vi "Get_All_Remote_SV_by_IP.vi"(8 "error in (no error)":errorcluster, 9 "timeout (30 s)":i32=30, 11 "IP Address":string="127.0.0.1") -> (0 "error out":errorcluster, 3 "Processes":T1(array[cluster]))   [LabVIEW 2016, in "DSC Remote SV Access.lvlib"]
doc: "This VI gets all the shared variables from a remote target.\n\nCreated By:\nRyan Pacini\n11/31/11"
uses:
  DSC Remote SV Access.lvlib
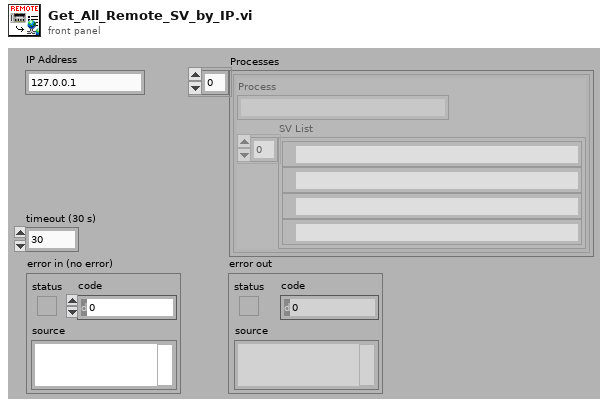
[diagram p1: front panel]
types:
  T1 = cluster{"Process":string, "SV List":refnum<k21>[]}[]
  T2 = cluster{string, "Shared Variable List":refnum<k21>[]}
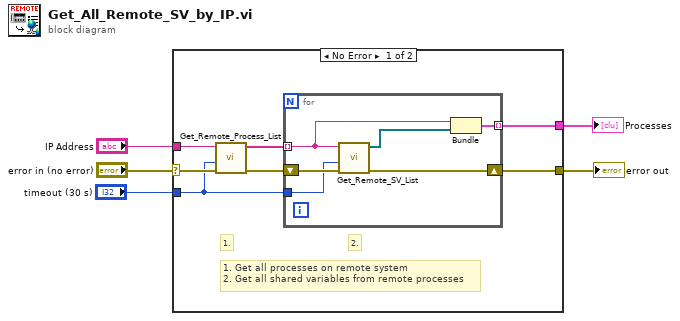
[diagram p0: block diagram]
diagram:
  n1 = case shown="No Error" "error in (no error)" {
    selector: "error in (no error)" -> [w7 w19]
    tunnel: [w10 _] -> w5
    tunnel: "IP Address" -> [w9 _]
    tunnel: [w8 w19] -> w3
    tunnel: "timeout (30 s)" -> [w6 _]
    frame No Error {
      # "1. Get all processes on remote system\n2. Get all shared variables from remote processes"
      # "2."
      # "1."
      n2 = call "Get_Remote_Process_List.vi"("error in (no error)"=w7, "timeout (30 s)"=w6, "IP Address"=w9) -> ("error out"=w12:errorcluster, "Process List (\\\\[IPAddress]\\[Process])"=w11:string[])  [unwired: 7 in]
      n3 = for {
        tunnel: w11 -> [w16] mode=indexing
        shift-right: [w17] -> w8
        shift-left: w12 -> [w18]
        tunnel: [w15] -> w10 mode=indexing
        tunnel: w6 -> [w14]
        n4 = call "Get_Remote_SV_List.vi"("error in (no error)"=w18, "timeout (30 s)"=w14, "Process (\\\\[IPAddress]\\[Process])"=w16) -> ("error out"=w17:errorcluster, "Shared Variable List"=w13:refnum<k21>[])  [unwired: 7 in]
        n5 = Bundle(w16, "Shared Variable List"=w13) -> (w15:T2)  [unwired: 1 in]
      }
    }
    frame Error {
    }
  }
  "Processes" <- w5
  "error out" <- w3
